vi "FWCS_TCPIP.vi"() -> ()   [LabVIEW 2018]
uses:
  RxTx/RxTx.lvclass
panel:
  in  "IP":string="200.131.64.49"
  in  "stop":bool
  out "error out 5":errorcluster
  out "error out 4":errorcluster
  out "error out 3":errorcluster
  out "error out 2":errorcluster
  in  "RxTx.lvclass 2":refnum<class "RxTx.lvclass">
  # "Channel 1 - TCPIP Communication"
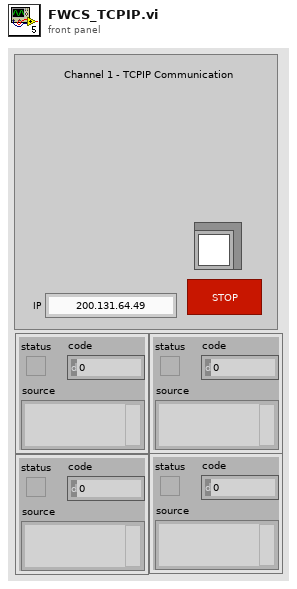
[diagram p1: front panel]
types:
  T1 = enum16{"Standard", "Buffered", "CRLF", "Immediate"}
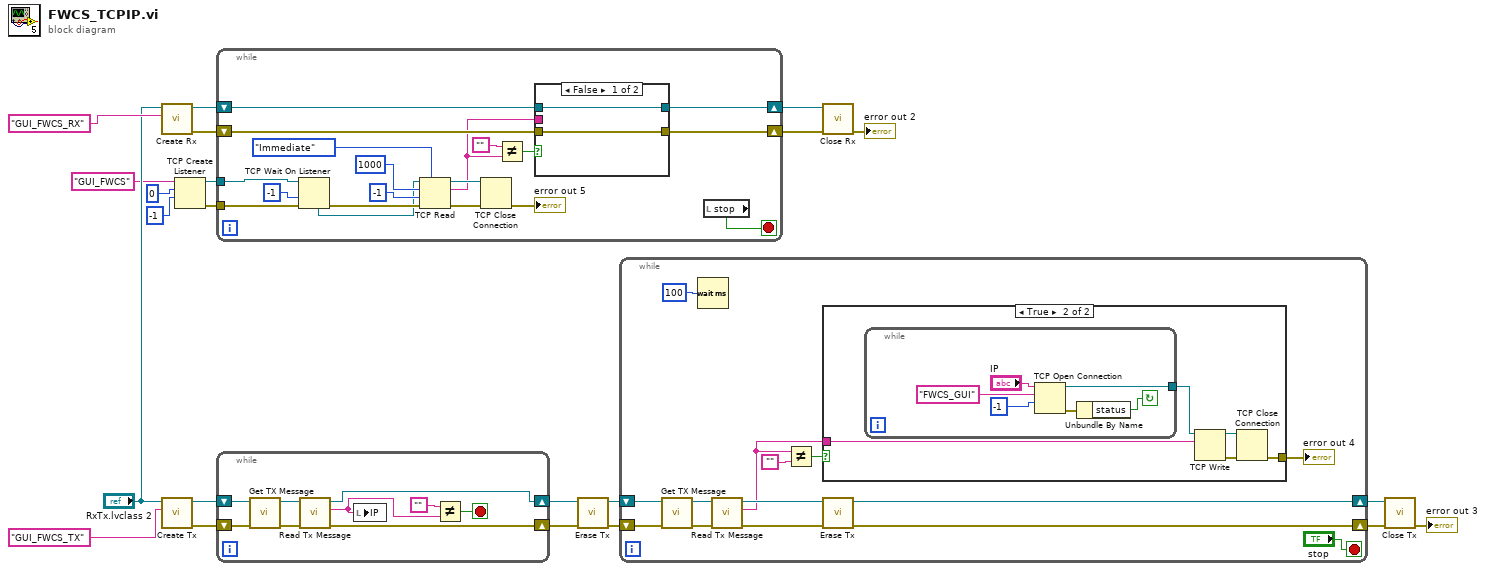
[diagram p0: block diagram]
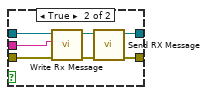
[diagram p3: hidden frame]
diagram:
  n1 = call "Create Rx.vi"("Reader Name"="GUI_FWCS_RX", "RxTx in"="RxTx.lvclass 2") -> ("error out"=w20:errorcluster, "RxTx out"=w21:refnum<class "RxTx.lvclass">)  [unwired: 8 in]
  n2 = call "Create Tx.vi"("Writer Name"="GUI_FWCS_TX" ("Reader Name"), "RxTx in"="RxTx.lvclass 2") -> ("error out"=w3:errorcluster, "RxTx out"=w4:refnum<class "RxTx.lvclass">)  [unwired: 8 in]
  n3 = TCP Create Listener(9:-1 ("timeout ms (25000)"), 10:u16 0 ("port"), 11:"GUI_FWCS" ("service name")) -> (0:w10:errorcluster, 3:w11:refnum<k5>)  [unwired: 2 in, 1 out]
  n4 = while {
    shift-right: [w36] -> w18
    shift-left: w20 -> [w41]
    shift-right: [w37] -> w19
    shift-left: w21 -> [w40]
    tunnel: w11 -> [w34]
    tunnel: w10 -> [w25]
    stop <- w35 stop-if-true
    n5 = TCP Wait On Listener(8:w25, 9:-1 ("timeout ms (wait forever: -1)"), 11:w34) -> (0:w29:errorcluster, 4:w24:refnum<k5>)  [unwired: 1 in, 3 out]
    n6 = TCP Read(connection ID=w24, bytes to read=1000, error in (no error)=w29, 7:T1."Immediate" ("mode (standard)"), 9:-1 ("timeout ms (25000)")) -> (connection ID out=w27:refnum<k5>, data out=w23:string, error out=w26:errorcluster)
    n7 = TCP Close Connection(connection ID=w27, error in (no error)=w26) -> (error out=→"error out 5":errorcluster)  [unwired: 1 in, 1 out]
    n8 = Not Equal?(x="", y=w23) -> (x != y?=w38:bool)
    n9 = case shown="False" w38 {
      tunnel: w41 -> [w42 w48]
      tunnel: w40 -> [w43 w47]
      tunnel: [w43 w46] -> w37
      tunnel: [w42 w45] -> w36
      tunnel: w23 -> [_ w44]
      frame False {
      }
      frame True {
        n10 = call "Write Rx Message.vi"("error in (no error)"=w48, "Rx Message"=w44, "RxTx in"=w47) -> ("error out"=w49:errorcluster, "RxTx out"=w50:refnum<class "RxTx.lvclass">)  [unwired: 7 in]
        n11 = call "Send RX Message.vi"("error in (no error)"=w49, "RxTx in"=w50) -> ("error out"=w45:errorcluster, "RxTx out"=w46:refnum<class "RxTx.lvclass">)  [unwired: 8 in]
      }
    }
    n12 = local read "stop"() -> (w35:bool)
  }
  n13 = while {
    shift-right: [w55] -> w7
    shift-left: w3 -> [w54]
    shift-right: [w53] -> w8
    shift-left: w4 -> [w52]
    stop <- w56 stop-if-true
    n14 = call "Get TX Message.vi"("error in (no error)"=w54, "RxTx in"=w52) -> ("error out"=w58:errorcluster, "RxTx out"=w59:refnum<class "RxTx.lvclass">)  [unwired: 8 in]
    n15 = call "Read Tx Message.vi"("error in (no error)"=w58, "RxTx in"=w59) -> ("error out"=w55:errorcluster, "Tx Message"=w51:string, "RxTx out"=w53:refnum<class "RxTx.lvclass">)  [unwired: 7 in]
    n16 = local write "IP"(w51) -> ()
    n17 = Not Equal?(x="", y=w51) -> (x != y?=w56:bool)
  }
  n18 = call "Erase Tx.vi"("error in (no error)"=w7, "RxTx in"=w8) -> ("error out"=w5:errorcluster, "RxTx out"=w6:refnum<class "RxTx.lvclass">)  [unwired: 8 in]
  n19 = while {
    shift-right: [w73] -> w16
    shift-left: w6 -> [w66]
    shift-right: [w72] -> w15
    shift-left: w5 -> [w65]
    stop <- "stop" stop-if-true
    n20 = call "Get TX Message.vi"("error in (no error)"=w65, "RxTx in"=w66) -> ("error out"=w71:errorcluster, "RxTx out"=w67:refnum<class "RxTx.lvclass">)  [unwired: 8 in]
    n21 = Wait (ms)(milliseconds to wait=u32 100) -> ()  [unwired: 1 out]
    n22 = call "Read Tx Message.vi"("error in (no error)"=w71, "RxTx in"=w67) -> ("error out"=w68:errorcluster, "Tx Message"=w60:string, "RxTx out"=w69:refnum<class "RxTx.lvclass">)  [unwired: 7 in]
    n23 = Not Equal?(x=w60, y="") -> (x != y?=w64:bool)
    n24 = case shown="True" w64 {
      tunnel: w60 -> [_ w78]
      tunnel: [_ w75] -> w63
      frame False {
      }
      frame True {
        n25 = while {
          tunnel: [w81] -> w77
          stop <- w84 continue-if-true
          n26 = TCP Open Connection(address="IP", remote port or service name="FWCS_GUI", timeout ms (60000)=-1 ("timeout")) -> (connection ID=w81:refnum<k5>, error out=w83:errorcluster)  [unwired: 2 in]
          n27 = Unbundle By Name(w83) -> ("status"=w84:bool)
        }
        n28 = TCP Write(connection ID=w77, data in=w78) -> (connection ID out=w74:refnum<k5>, error out=w76:errorcluster)  [unwired: 2 in, 1 out]
        n29 = TCP Close Connection(connection ID=w74, error in (no error)=w76) -> (error out=w75:errorcluster)  [unwired: 1 in, 1 out]
      }
    }
    "error out 4" <- w63
    n30 = call "Erase Tx.vi"("error in (no error)"=w68, "RxTx in"=w69) -> ("error out"=w72:errorcluster, "RxTx out"=w73:refnum<class "RxTx.lvclass">)  [unwired: 8 in]
  }
  n31 = call "Close Rx.vi"("error in (no error)"=w18, "RxTx in"=w19) -> ("error out"=→"error out 2":errorcluster)  [unwired: 8 in, 1 out]
  n32 = call "Close Tx.vi"("error in (no error)"=w15, "RxTx in"=w16) -> ("error out"=→"error out 3":errorcluster)  [unwired: 8 in, 1 out]
